vi "sendCmdFromTcpClient.vi"(8 "error in (no error)":errorcluster, 11 "connection ID in":refnum<k5>) -> (0 "error out":errorcluster, 2 "ack received":string[](array[string]), 3 "connection ID out":refnum<k5>)   [LabVIEW 2018]
doc: "Generate commands as JSON packets and send them to TCP server, and then read the response from TCP server."
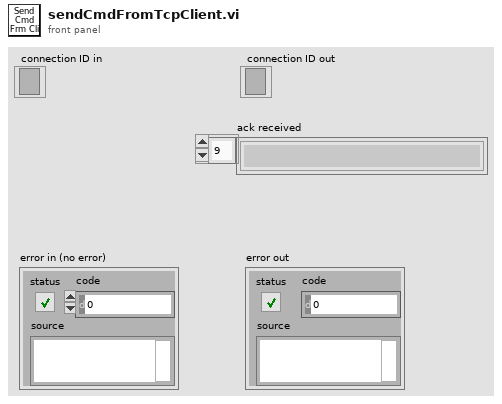
[diagram p1: front panel]
types:
  T1 = enum16{"Standard", "Buffered", "CRLF", "Immediate"}
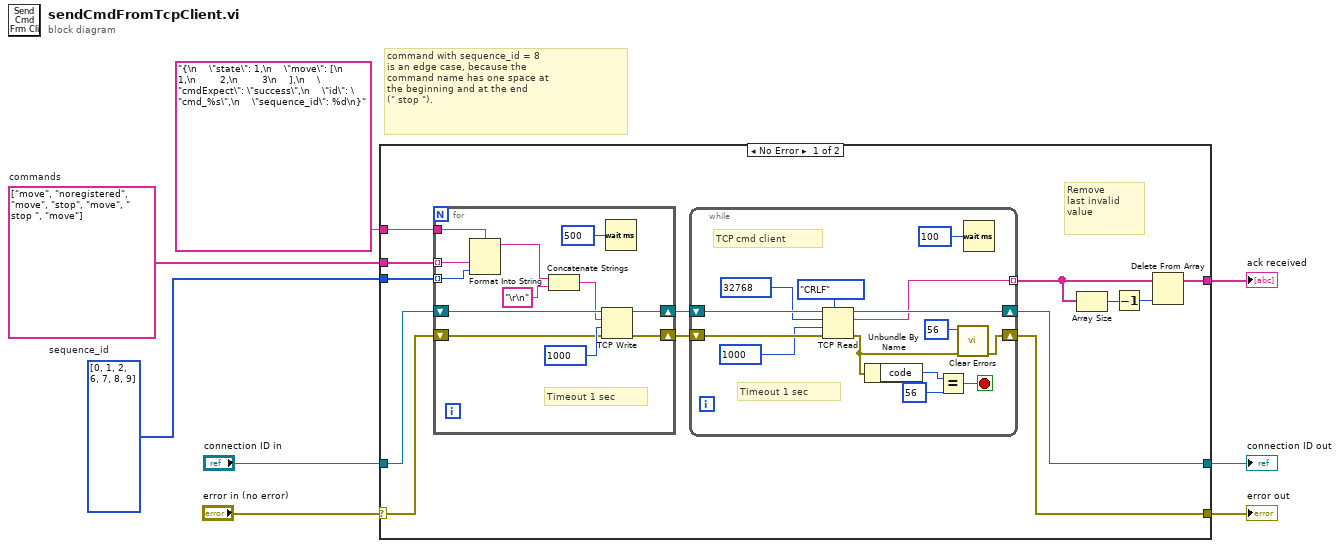
[diagram p0: block diagram]
diagram:
  w1 = i32[] [0, 1, 2, 6, 7, 8, 9]  # sequence_id
  w2 = string[] ["move", "noregistered", "move", "stop", "move", " stop ", "move"]  # commands
  # "command with sequence_id = 8\nis an edge case, because the\ncommand name has one space at\nthe beginning and at the end\n(\" stop \")."
  n1 = case shown="No Error" "error in (no error)" {
    selector: "error in (no error)" -> [w20 w49]
    tunnel: [w21 w48] -> w8
    tunnel: [w19 w49] -> w6
    tunnel: [w18 _] -> w5
    tunnel: "connection ID in" -> [w17 w48]
    tunnel: "{\n    \"state\": 1,\n    \"move\": [\n        1,\n        2,\n        3\n    ],\n    \"cmdExpect\": \"success\",\n    \"id\": \"cmd_%s\",\n    \"sequence_id\": %d\n}" ("Display") -> [w14 _]
    tunnel: w2 -> [w13 _]
    tunnel: w1 -> [w12 _]
    frame No Error {
      # "Remove \nlast invalid \nvalue"
      n2 = for {
        shift-right: [w46] -> w16
        shift-left: w20 -> [w41]
        shift-right: [w43] -> w15
        shift-left: w17 -> [w42]
        tunnel: w14 -> [w39]
        tunnel: w13 -> [w38] mode=indexing
        tunnel: w12 -> [w37] mode=indexing
        # "Timeout 1 sec"
        n3 = Format Into String(format string=w39, w38, w37) -> (resulting string=w36:string)  [unwired: 2 in, 1 out]
        n4 = Concatenate Strings(w36, "\r\n" ("string")) -> (w40:string)
        n5 = TCP Write(connection ID=w42, data in=w40, error in (no error)=w41, 9:1000 ("timeout ms (25000)")) -> (connection ID out=w43:refnum<k5>, error out=w46:errorcluster)  [unwired: 1 out]
        n6 = Wait (ms)(milliseconds to wait=u32 500) -> ()  [unwired: 1 out]
      }
      n7 = while {
        tunnel: [w22] -> w11 mode=indexing
        shift-right: [w23] -> w19
        shift-left: w16 -> [w32]
        shift-right: [w29] -> w21
        shift-left: w15 -> [w33]
        stop <- w26 stop-if-true
        # "TCP cmd client"
        # "Timeout 1 sec"
        n8 = TCP Read(connection ID=w33, bytes to read=32768, error in (no error)=w32, 7:T1."CRLF" ("mode (standard)"), 9:1000 ("timeout ms (25000)")) -> (connection ID out=w29:refnum<k5>, data out=w22:string, error out=w25:errorcluster)
        n9 = Unbundle By Name(w25) -> ("code"=w28:i32)
        n10 = Equal?(x=w28, y=56) -> (x = y?=w26:bool)
        n11 = call <vilib>:"Clear Errors.vi"("error in (no error)"=w25, "specific error code to clear (0: all)"=56) -> ("error out"=w23:errorcluster)  [unwired: 4 in, 1 out]
        n12 = Wait (ms)(milliseconds to wait=u32 100) -> ()  [unwired: 1 out]
      }
      n13 = Array Size(array=w11) -> (size(s)=w10:i32)
      n14 = Decrement(x=w10) -> (x-1=w9:i32)
      n15 = Delete From Array(array=w11, index=w9) -> (array with subset deleted=w18:string[])  [unwired: 1 in, 1 out]
    }
    frame Error {
    }
  }
  "connection ID out" <- w8
  "error out" <- w6
  "ack received" <- w5
